vi "Create Pattern Script(Data).vi"(7 "Data Type":T1, 8 "error in (no error)":errorcluster, 10 "Data":u16, 11 "SPI 4W Pattern Creator in":refnum<class "SPI 4W Pattern Creator.lvclass">) -> (0 "error out":errorcluster, 2 "String":string, 3 "SPI 4W Pattern Creator out":refnum<class "SPI 4W Pattern Creator.lvclass">)   [LabVIEW 2018, in "SPI 4W Pattern Creator.lvlib" / "SPI 4W Pattern Creator.lvclass"]
uses:
  SPI 4W Pattern Creator.lvclass
  Protocols/SPI Root Pattern Creator.lvlibp/Plugins/SouceCode/SPI_Pattern Creator/SPI Root/Data Type.ctl
  Interfaces/Protocol Interface.lvlibp/Interfaces/Protocol Interface/Pin State.ctl
  Interfaces/Protocol Interface.lvlibp/Interfaces/Protocol Interface/Protocol Interface.lvclass
  Protocols/SPI Root Pattern Creator.lvlibp/Plugins/SouceCode/SPI_Pattern Creator/SPI Root/SPI Root Pattern Creator.lvclass
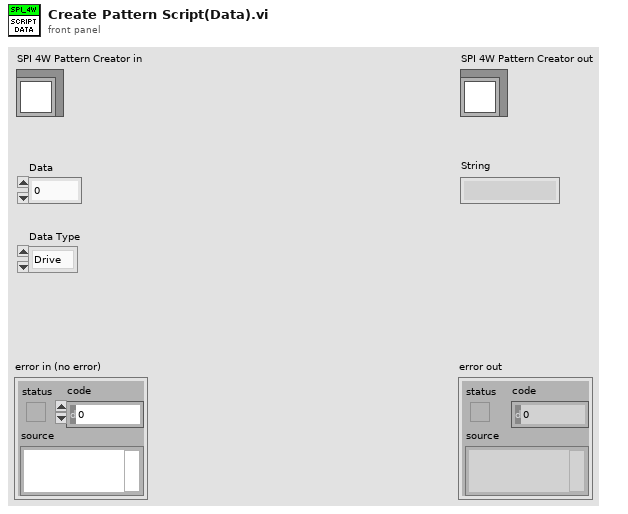
[diagram p1: front panel]
types:
  T1 = typedef "SPI Root Pattern Creator.lvlibp/SPI Root Pattern Creator.lvclass/Data Type.ctl" = enum16{"Drive", "Compare", "Read"}
  T2 = typedef "Protocol Interface.lvlibp/Protocol Interface.lvclass/Pin State.ctl" = enum16{"0", "1", "L", "H", "X", "V", "D", "M"}
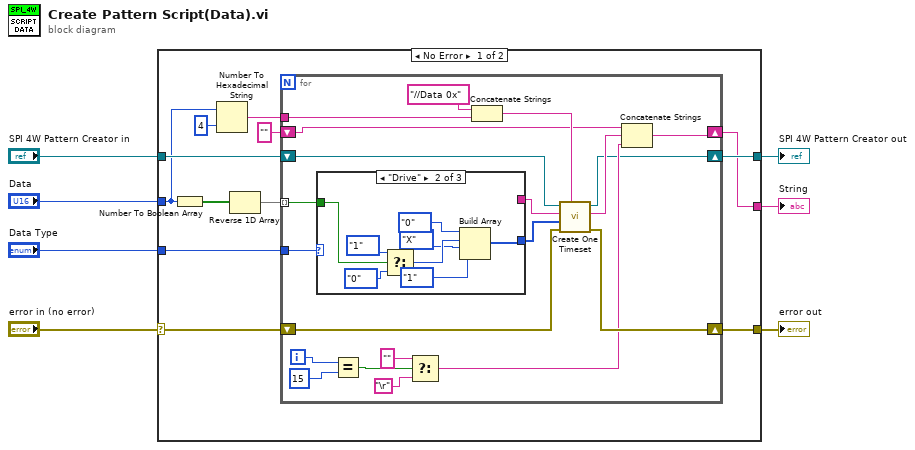
[diagram p0: block diagram]
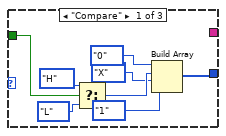
[diagram p2: hidden frame]
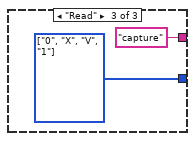
[diagram p3: hidden frame]
diagram:
  n1 = case shown="No Error" "error in (no error)" {
    selector: "error in (no error)" -> [w15 w59]
    tunnel: "SPI 4W Pattern Creator in" -> [w16 w58]
    tunnel: "Data" -> [w14 _]
    tunnel: "Data Type" -> [w17 _]
    tunnel: [w10 w58] -> w4
    tunnel: [w9 _] -> w3
    tunnel: [w8 w59] -> w2
    frame No Error {
      n2 = Number To Boolean Array(number=w14) -> (Boolean array=w19:bool[])
      n3 = Number To Hexadecimal String(1:i16 4 ("width (-)"), 2:w14) -> (0:w12:string)
      n4 = Reverse 1D Array(array=w19) -> (reversed array=w18:bool[])
      n5 = for {
        tunnel: w18 -> [w35] mode=indexing
        tunnel: w17 -> [w39]
        shift-right: [w20] -> w10
        shift-left: w16 -> [w36]
        shift-right: [w33] -> w8
        shift-left: w15 -> [w34]
        tunnel: w12 -> [w32]
        shift-right: [w23] -> w9
        shift-left: "" -> [w22]
        i -> [w29]
        n6 = case shown="\"Drive\"" w39 {
          tunnel: [w42 w50 w57] -> w38
          tunnel: [_ _ "capture"] -> w37
          tunnel: w35 -> [w46 w54 _]
          frame "Compare" {
            n7 = Select(t=Pin_State."H" ("PinState"), s=w46, f=Pin_State."L" ("PinState")) -> (s? t:f=w41:T2)
            n8 = Build Array(Pin_State."0" ("PinState"), w41, Pin_State."X" ("PinState"), Pin_State."1" ("element")) -> (w42:T2[])
          }
          frame "Drive" {
            n9 = Select(t=Pin_State."1" ("PinState"), s=w54, f=Pin_State."0" ("PinState")) -> (s? t:f=w49:T2)
            n10 = Build Array(Pin_State."0" ("PinState"), w49, Pin_State."X" ("PinState"), Pin_State."1" ("element")) -> (w50:T2[])
          }
          frame "Read" {
            w57 = T2[] [enum."0", enum."X", enum."V", enum."1"] items=["0", "1", "L", "H", "X", "V", "D", "M"]
          }
        }
        n11 = Equal?(x=w29, y=15) -> (x = y?=w27:bool)
        n12 = Select(t="", s=w27, f="\r") -> (s? t:f=w21:string)
        n13 = Concatenate Strings("//Data 0x" ("string"), w32) -> (w30:string)
        n14 = call-dynamic "Create One Timeset.vi"("Notes"=w30, "error in (no error)"=w34, "PinStates"=w38, "OpCode"=w37, "SPI 4W Pattern Creator in"=w36) -> ("error out"=w33:errorcluster, "String  out"=w24:string, "SPI 4W Pattern Creator out"=w20:refnum<class "SPI 4W Pattern Creator.lvclass">)  [unwired: 4 in]
        n15 = Concatenate Strings(w22, w24, w21) -> (w23:string)
      }
    }
    frame Error {
    }
  }
  "error out" <- w2
  "SPI 4W Pattern Creator out" <- w4
  "String" <- w3
